vi "CloseReferences.vi"(8 "error in (no error)":errorcluster) -> (0 "error out":errorcluster)   [LabVIEW 2013, in "ProjectHandler.lvlib"]
uses:
  ProjectHandler.lvlib
  RefNums.vi
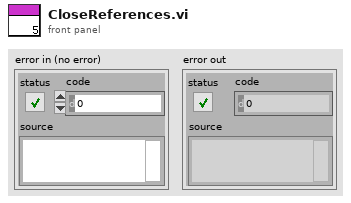
[diagram p1: front panel]
types:
  T1 = cluster{"App":refnum<vi>, "Project":refnum<vi>, "My Computer":refnum<vi>}
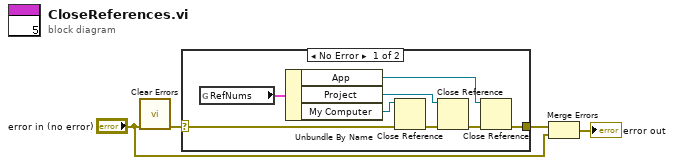
[diagram p0: block diagram]
diagram:
  n1 = call <vilib>:"Clear Errors.vi"("error in (no error)"="error in (no error)") -> ("error out"=w4:errorcluster)  [unwired: 6 in]
  n2 = case shown="No Error" w4 {
    selector: w4 -> [w8 w13]
    tunnel: [w5 w13] -> w2
    frame No Error {
      n3 = global read "RefNums.vi" "RefNums"() -> (w12:T1)
      n4 = Unbundle By Name(w12) -> ("App"=w11:refnum<vi>, "Project"=w10:refnum<vi>, "My Computer"=w9:refnum<vi>)
      n5 = Close Reference(reference=w9, error in (no error)=w8) -> (error out=w7:errorcluster)
      n6 = Close Reference(reference=w10, error in (no error)=w7) -> (error out=w6:errorcluster)
      n7 = Close Reference(reference=w11, error in (no error)=w6) -> (error out=w5:errorcluster)
    }
    frame Error {
    }
  }
  n8 = Merge Errors(w2, "error in (no error)") -> (→"error out":errorcluster)
